vi "Periodic Tasks.vi"(11 "error in":errorcluster) -> ()   [LabVIEW 2017]
doc: "This VI runs in parallel to other tasks. It can contain as many user-defined periodic loops as you need. These can carry out PID or other sorts of timed response."
uses:
  <vilib>/Rock Robotics/Network Tables/NT Write String Array.vi
panel:
  in  "error in (no error)":errorcluster
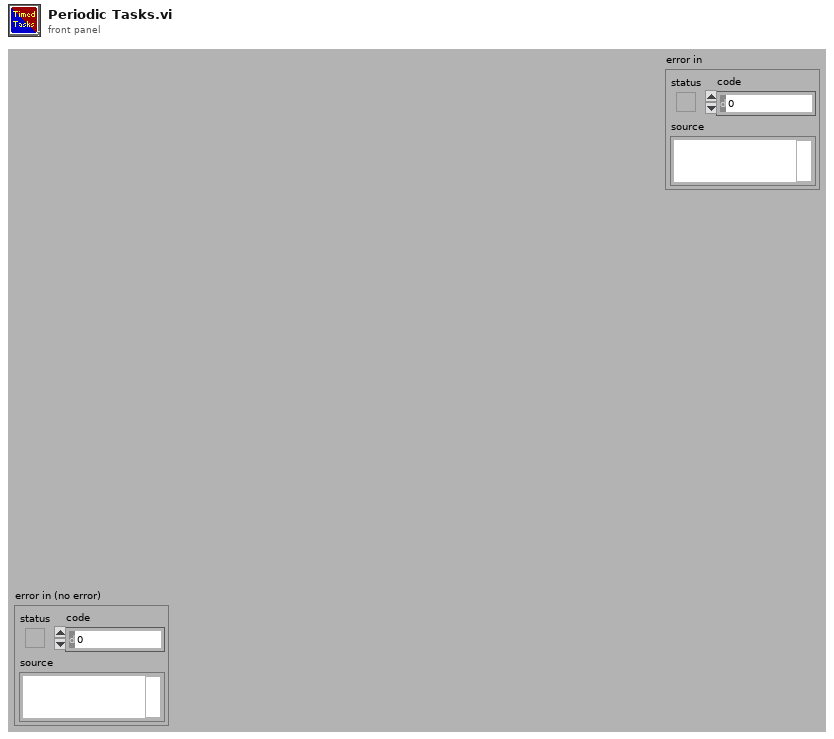
[diagram p1: front panel]
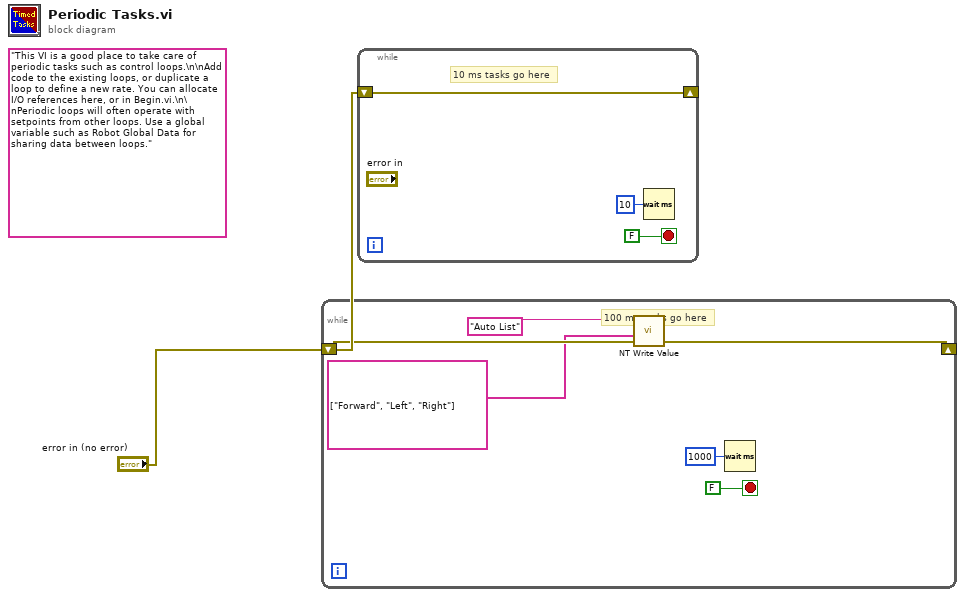
[diagram p0: block diagram]
diagram:
  (unwired) "This VI is a good place to take care of periodic tasks such as control loops.\n\nAdd code to the existing loops, or duplicate a loop to define a new rate. You can allocate I/O references here, or in Begin.vi.\n\nPeriodic loops will often operate with setpoints from other loops. Use a global variable such as Robot Global Data for sharing data between loops."
  n1 = while {
    shift-right: [w4] -> _
    shift-left: "error in (no error)" -> [w4]
    stop <- FALSE stop-if-true
    # "100 ms tasks go here"
    n2 = call-poly <vilib>:"NT Write Value.vi"("String Array"=string[] ["Forward", "Left", "Right"], "Name"="Auto List") -> ()  [unwired: 9 in, 1 out]
    n3 = Wait (ms)(milliseconds to wait=u32 1000) -> ()  [unwired: 1 out]
  }
  n4 = while {
    shift-right: [w7] -> _
    shift-left: "error in (no error)" -> [w7]
    stop <- FALSE stop-if-true
    # "10 ms tasks go here"
    n5 = Wait (ms)(milliseconds to wait=u32 10) -> ()  [unwired: 1 out]
  }
